vi "GetArrayFmTxtFile.vi"(2 "error in":errorcluster, 3 "LineNo.":i32, 4 "TextFile":path=path "C:/Users/TTUHEP/Documents/LabVIEW/Data/AssemblyIO_logs/BaseplatePositions.txt") -> (0 "error out":errorcluster, 1 "Array":dbl[](array[numeric]))   [LabVIEW 2021]
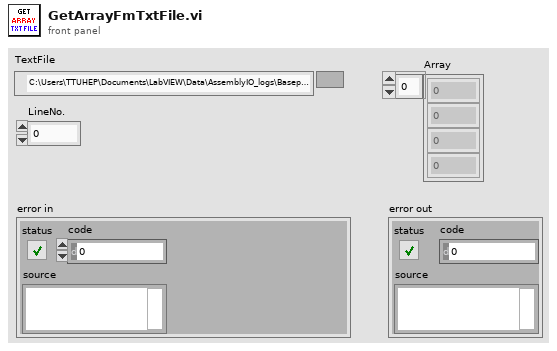
[diagram p1: front panel]
types:
  T1 = enum16{"open", "replace", "create", "open or create", "replace or create", "replace or create with confirmation"}
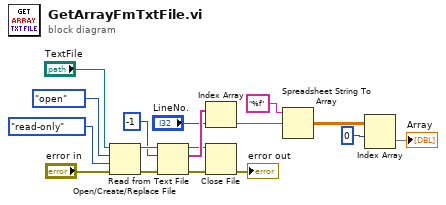
[diagram p0: block diagram]
diagram:
  n1 = Open/Create/Replace File(file path (use dialog)="TextFile", error in="error in", operation (0:open)=T1."open", access (0:read/write)=enum16{"read/write", "read-only", "write-only"}."read-only") -> (refnum out=w14:refnum<file>, error out=w15:errorcluster)  [unwired: 2 in, 1 out]
  n2 = Read from Text File(file (use dialog)=w14, count=-1, error in=w15) -> (refnum out=w3:refnum<file>, text=w11:string[], error out=w2:errorcluster)  [unwired: 1 in, 1 out]
  n3 = Index Array(array=w11, index="LineNo.") -> (element=w8:string)
  n4 = Close File(refnum=w3, error in=w2) -> (error out=→"error out":errorcluster)  [unwired: 1 out]
  n5 = Spreadsheet String To Array(format string="%f" ("spreadsheet string"), spreadsheet string=w8) -> (array=w6:dbl[][])  [unwired: 2 in]
  n6 = Index Array(array=w6, index (row)=0) -> (element=→"Array":dbl[])  [unwired: 1 in]
